vi "Drive.vi"(0 "Enum":enum16{"Start", "Run", "End"}(ring), 5 "Left Primary":dbl, 7 "Left Secondary":dbl, 9 "Right Primary":dbl, 11 "Right Secondary":dbl) -> ()   [LabVIEW 2014]
uses:
  <vilib>/Rock Robotics/SystemInterfaces/DIO/FPGA_DIOPWMChannel.ctl
  <vilib>/Rock Robotics/WPI/MotorControl/WPI_MotorControlOpen Talon.vi
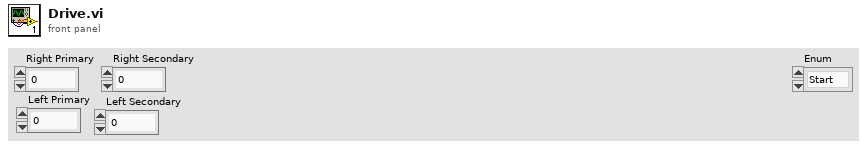
[diagram p1: front panel]
types:
  T1 = typedef "FPGA_DIOPWMChannel.ctl" = enum8{"PWM 0", "PWM 1", "PWM 2", "PWM 3", "PWM 4", "PWM 5", "PWM 6", "PWM 7", "PWM 8", "PWM 9", "PWM MXP 0", "PWM MXP 1", "PWM MXP 2", "PWM MXP 3", "PWM MXP 4", "PWM MXP 5", "PWM MXP 6", "PWM MXP 7", "PWM MXP 8", "PWM MXP 9", "Invalid"}
  T2 = typedef "WPI_MotorControlDeviceRef.ctl" = cluster{"DeviceStatus":errorcluster, "Type":T3, "PWM":cluster{"Controller":T4, "PWM Channel":T1, "DeadBand":T5}, "CAN":cluster{"Device Number":u8, "Control Mode":T6, "Semaphore":T7, "Max Vout":dbl, "TalonSRX Control Mode":T8}, "Invert":bool, "TransformRef":T9, "InvTransformRef":T9}
  T3 = typedef "WPI_MotorControlType.ctl" = enum16{"PWM", "CAN", "CANTalonSRX"}
  T4 = typedef "FPGA_TypedefDigitalModule.ctl" = enum16{"Controller 1"}
  T5 = typedef "WPI_PWMDeadband.ctl" = cluster{"Name":string, "maxPositivePwm":i32, "minPositivePwm":i32, "centerPwm":i32, "maxNegativePwm":i32, "minNegativePwm":i32, "angularRange":u16}
  T6 = typedef "WPI_CANJaguar_ControlMode.ctl" = enum8{"Percent VBus", "Current", "Speed", "Position", "Voltage"}
  T7 = typedef "Semaphore RefNum" = refnum<k1>
  T8 = typedef "WPI_CANTalonSRX_APIControlMode.ctl" = enum8{"Percent VBus", "Speed", "Position", "Slave", "Unchanged / Invalid"}
  T9 = typedef "WPI_PWMTransform_ConPane.ctl" = refnum<vi>
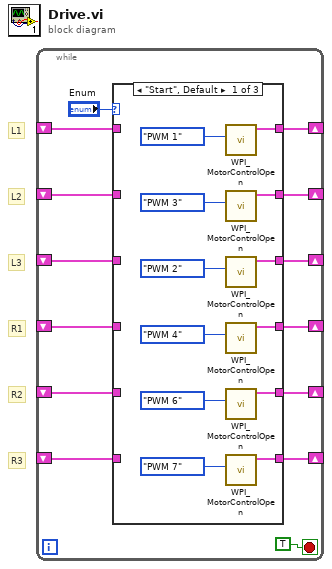
[diagram p0: block diagram]
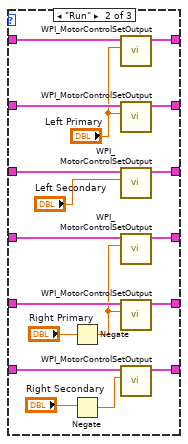
[diagram p2: hidden frame]
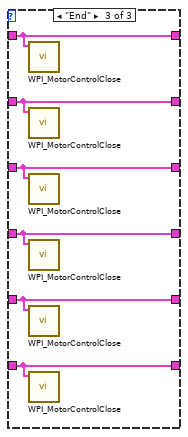
[diagram p3: hidden frame]
diagram:
  # "R3"
  # "R2"
  # "R1"
  # "L3"
  # "L2"
  # "L1"
  n1 = while {
    shift-right: [w12] -> _
    shift-left: _ -> [w1]
    shift-right: [w11] -> _
    shift-left: _ -> [w2]
    shift-right: [w10] -> _
    shift-left: _ -> [w3]
    shift-right: [w9] -> _
    shift-left: _ -> [w4]
    shift-right: [w8] -> _
    shift-left: _ -> [w5]
    shift-right: [w7] -> _
    shift-left: _ -> [w6]
    stop <- TRUE stop-if-true
    n2 = case shown="\"Start\", Default" "Enum" {
      tunnel: [w26 w43 w45] -> w12
      tunnel: [w25 w41 w46] -> w11
      tunnel: [w24 w39 w47] -> w10
      tunnel: [w23 w37 w48] -> w9
      tunnel: [w22 w35 w49] -> w8
      tunnel: [w21 w33 w50] -> w7
      tunnel: w6 -> [_ w34 w50]
      tunnel: w5 -> [_ w36 w49]
      tunnel: w4 -> [_ w38 w48]
      tunnel: w3 -> [_ w40 w47]
      tunnel: w2 -> [_ w42 w46]
      tunnel: w1 -> [_ w44 w45]
      frame "Start", Default {
        n3 = call-poly <vilib>:"WPI_MotorControlOpen.vi"("PWM Channel"=FPGA_DIOPWMChannel."PWM 1") -> ("MotorControlDeviceRef"=w26:T2)  [unwired: 9 in, 1 out]
        n4 = call-poly <vilib>:"WPI_MotorControlOpen.vi"("PWM Channel"=FPGA_DIOPWMChannel."PWM 3") -> ("MotorControlDeviceRef"=w25:T2)  [unwired: 9 in, 1 out]
        n5 = call-poly <vilib>:"WPI_MotorControlOpen.vi"("PWM Channel"=FPGA_DIOPWMChannel."PWM 2") -> ("MotorControlDeviceRef"=w24:T2)  [unwired: 9 in, 1 out]
        n6 = call-poly <vilib>:"WPI_MotorControlOpen.vi"("PWM Channel"=FPGA_DIOPWMChannel."PWM 4") -> ("MotorControlDeviceRef"=w23:T2)  [unwired: 9 in, 1 out]
        n7 = call-poly <vilib>:"WPI_MotorControlOpen.vi"("PWM Channel"=FPGA_DIOPWMChannel."PWM 6") -> ("MotorControlDeviceRef"=w22:T2)  [unwired: 9 in, 1 out]
        n8 = call-poly <vilib>:"WPI_MotorControlOpen.vi"("PWM Channel"=FPGA_DIOPWMChannel."PWM 7") -> ("MotorControlDeviceRef"=w21:T2)  [unwired: 9 in, 1 out]
      }
      frame "Run" {
        n9 = Negate(x="Right Primary") -> (-x=w32:dbl)
        n10 = Negate(x="Right Secondary") -> (-x=w28:dbl)
        n11 = call <vilib>:"WPI_MotorControlSetOutput.vi"("Output"="Left Primary", "MotorControlDevRef"=w44) -> ("MotorControlDevRef"=w43:T2)  [unwired: 7 in, 2 out]
        n12 = call <vilib>:"WPI_MotorControlSetOutput.vi"("Output"="Left Primary", "MotorControlDevRef"=w42) -> ("MotorControlDevRef"=w41:T2)  [unwired: 7 in, 2 out]
        n13 = call <vilib>:"WPI_MotorControlSetOutput.vi"("Output"="Left Secondary", "MotorControlDevRef"=w40) -> ("MotorControlDevRef"=w39:T2)  [unwired: 7 in, 2 out]
        n14 = call <vilib>:"WPI_MotorControlSetOutput.vi"("Output"=w32, "MotorControlDevRef"=w38) -> ("MotorControlDevRef"=w37:T2)  [unwired: 7 in, 2 out]
        n15 = call <vilib>:"WPI_MotorControlSetOutput.vi"("Output"=w32, "MotorControlDevRef"=w36) -> ("MotorControlDevRef"=w35:T2)  [unwired: 7 in, 2 out]
        n16 = call <vilib>:"WPI_MotorControlSetOutput.vi"("Output"=w28, "MotorControlDevRef"=w34) -> ("MotorControlDevRef"=w33:T2)  [unwired: 7 in, 2 out]
      }
      frame "End" {
        n17 = call <vilib>:"WPI_MotorControlClose.vi"("MotorControlDevRef"=w45) -> ()  [unwired: 10 in, 1 out]
        n18 = call <vilib>:"WPI_MotorControlClose.vi"("MotorControlDevRef"=w46) -> ()  [unwired: 10 in, 1 out]
        n19 = call <vilib>:"WPI_MotorControlClose.vi"("MotorControlDevRef"=w47) -> ()  [unwired: 10 in, 1 out]
        n20 = call <vilib>:"WPI_MotorControlClose.vi"("MotorControlDevRef"=w48) -> ()  [unwired: 10 in, 1 out]
        n21 = call <vilib>:"WPI_MotorControlClose.vi"("MotorControlDevRef"=w49) -> ()  [unwired: 10 in, 1 out]
        n22 = call <vilib>:"WPI_MotorControlClose.vi"("MotorControlDevRef"=w50) -> ()  [unwired: 10 in, 1 out]
      }
    }
  }
